vi "Name.vi"(11 "Condition Value in":refnum<class "Condition Value.lvclass">) -> (2 "Name":string)   [LabVIEW 2020, in "VolatusSeq.lvlib" / "Condition Value.lvclass"]
uses:
  Condition Value.lvclass
  Condition Value.lvclass/Condition Value.ctl
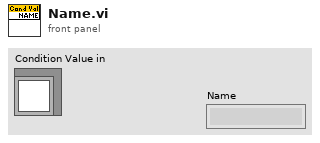
[diagram p1: front panel]
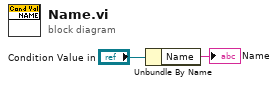
[diagram p0: block diagram]
diagram:
  n1 = Unbundle By Name("Condition Value in") -> ("Name"=→"Name":string)
